vi "Read Source Actor.vi"(8 "error in (no error)":errorcluster, 11 "Error Display Actor in":refnum<class "Error Display Actor.lvclass">) -> (0 "error out":errorcluster, 2 "Source Actor":string, 3 "Error Display Actor out":refnum<class "Error Display Actor.lvclass">)   [LabVIEW 2020, in "ViewableActor.lvlib" / "Error Display Actor.lvclass"]
uses:
  Error Display Actor.lvclass
  Error Display Actor.lvclass/Error Display Actor.ctl
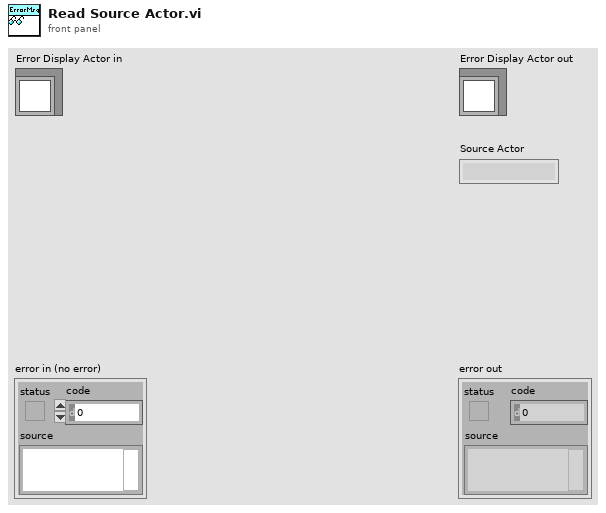
[diagram p1: front panel]
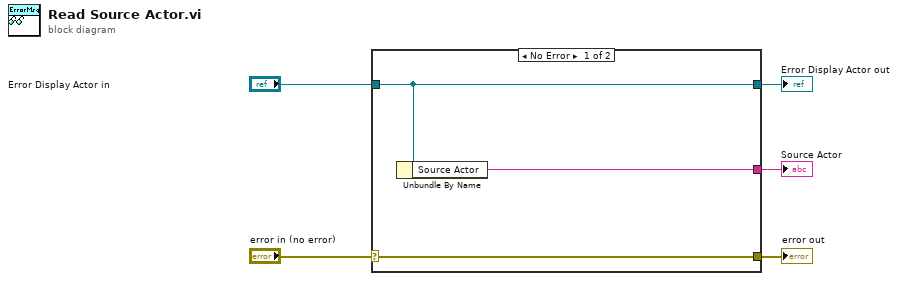
[diagram p0: block diagram]
diagram:
  n1 = case shown="No Error" "error in (no error)" {
    selector: "error in (no error)" -> [w8 w9]
    tunnel: [w8 w9] -> w4
    tunnel: [w7 w10] -> w2
    tunnel: "Error Display Actor in" -> [w7 w10]
    tunnel: [w6 _] -> w1
    frame No Error {
      n2 = Unbundle By Name(w7) -> ("Source Actor"=w6:string)
    }
    frame Error {
    }
  }
  "error out" <- w4
  "Error Display Actor out" <- w2
  "Source Actor" <- w1
